vi "Queue Example.vi"() -> ()   [LabVIEW 2011]
panel:
  out "element 3":string
  out "element 2":string
  out "element":string
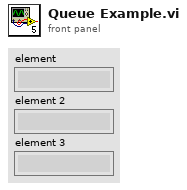
[diagram p1: front panel]
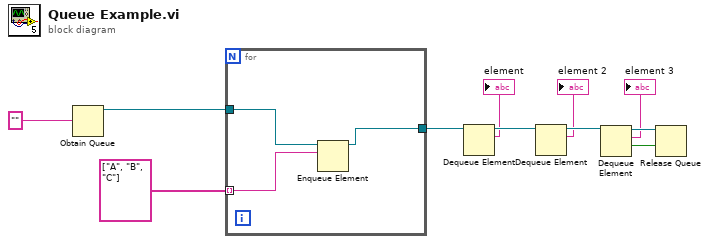
[diagram p0: block diagram]
diagram:
  n1 = Obtain Queue(element data type="") -> (queue out=w9:refnum<queue>)  [unwired: 4 in, 2 out]
  n2 = for {
    tunnel: string[] ["A", "B", "C"] -> [w13] mode=indexing
    tunnel: w9 -> [w14]
    tunnel: [w12] -> w8
    n3 = Enqueue Element(queue=w14, element=w13) -> (queue out=w12:refnum<queue>)  [unwired: 2 in, 2 out]
  }
  n4 = Dequeue Element(queue=w8) -> (queue out=w5:refnum<queue>, element=→"element":string)  [unwired: 2 in, 2 out]
  n5 = Dequeue Element(queue=w5) -> (queue out=w4:refnum<queue>, element=→"element 2":string)  [unwired: 2 in, 2 out]
  n6 = Dequeue Element(queue=w4) -> (queue out=w7:refnum<queue>, element=→"element 3":string, timed out?=w6:bool)  [unwired: 2 in, 1 out]
  n7 = Release Queue(queue=w7, force destroy? (F)=w6) -> ()  [unwired: 1 in, 3 out]
